vi "GCS3 Begin Block.vi"(0 "Line to Parse":string, 5 "error in":errorcluster, 6 "Expected GCS 3.0 Block Name":string) -> (14 "GCS 3.0 Block Name":string, 15 "Array of GCS 3.0 Block Entries":string[](array[string]), 16 "Is GCS 3.0 Block?":bool, 19 "error out":errorcluster)   [LabVIEW 2026]
uses:
  <vilib>/regexp/Match Regular Expression.xnode
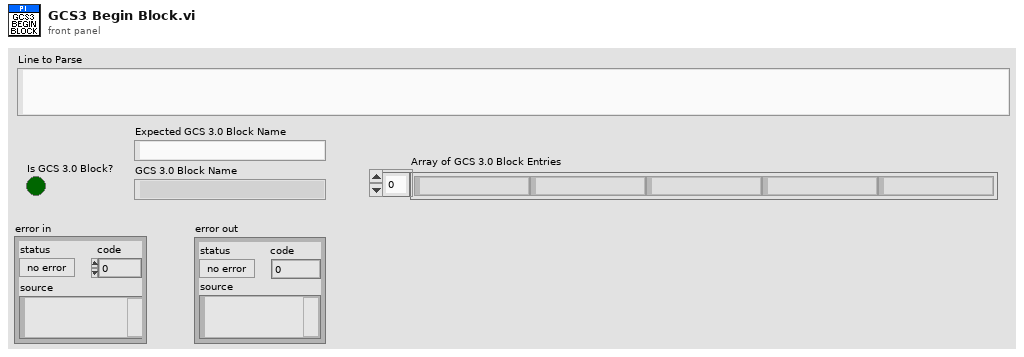
[diagram p1: front panel]
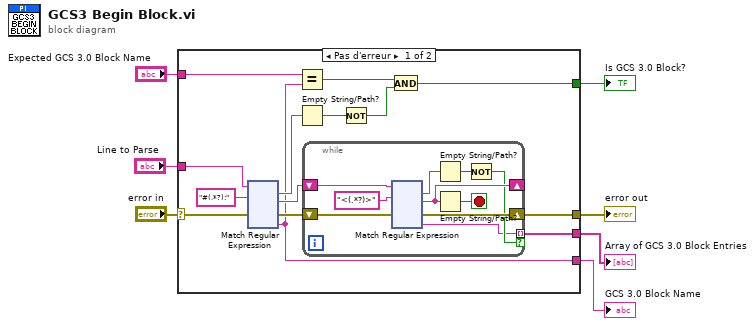
[diagram p0: block diagram]
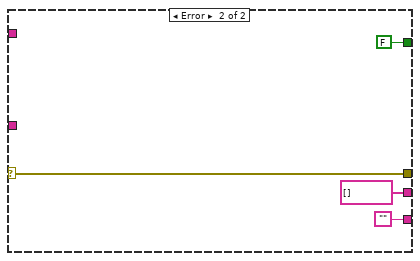
[diagram p2: hidden frame]
diagram:
  n1 = case shown="Pas d'erreur" "error in" {
    selector: "error in" -> [w20 w273]
    tunnel: [w15 w273] -> w6
    tunnel: "Line to Parse" -> [w21 _]
    tunnel: [w9 FALSE] -> w4
    tunnel: [w8 ""] -> w3
    tunnel: [w14 string[] [] ("Array of GCS 3.0 Block Entries")] -> w2
    tunnel: "Expected GCS 3.0 Block Name" -> [w13 _]
    frame No Error {
      n2 = xnode "Match Regular Expression"("chaîne en entrée"=w21, "expression régulière"="#(.*?):" ("regular expression"), "entrée d'erreur"=w20) -> ("toute l'expression"=w12:string, "après la correspondance"=w17:string, "sortie d'erreur"=w16:errorcluster, "correspondance partielle 1"=w8:string)  [unwired: 3 in, 2 out]
      n3 = Equal?(x=w13, y=w8) -> (x = y?=w10:bool)
      n4 = Empty String/Path?(string/path=w12) -> (empty?=w18:bool)
      n5 = while {
        shift-right: [w26] -> _
        shift-left: w17 -> [w31]
        shift-right: [w29] -> w15
        shift-left: w16 -> [w30]
        tunnel: [w22] -> w14 mode=indexing if=w23
        stop <- w27 stop-if-true
        n6 = xnode "Match Regular Expression"("chaîne en entrée"=w31, "expression régulière"="<(.*?)>" ("regular expression"), "entrée d'erreur"=w30) -> ("toute l'expression"=w25:string, "après la correspondance"=w26:string, "sortie d'erreur"=w29:errorcluster, "correspondance partielle 1"=w22:string)  [unwired: 3 in, 2 out]
        n7 = Empty String/Path?(string/path=w25) -> (empty?=w24:bool)
        n8 = Empty String/Path?(string/path=w26) -> (empty?=w27:bool)
        n9 = Not(x=w24) -> (.not. x?=w23:bool)
      }
      n10 = Not(x=w18) -> (.not. x?=w11:bool)
      n11 = And(x=w10, y=w11) -> (x .and. y?=w9:bool)
    }
    frame Error {
    }
  }
  "error out" <- w6
  "Is GCS 3.0 Block?" <- w4
  "Array of GCS 3.0 Block Entries" <- w2
  "GCS 3.0 Block Name" <- w3
